vi "lvEtherbone.error_handler.vi"(2 "eb_status":T1, 5 "error in":errorcluster) -> (19 "error out":errorcluster)   [LabVIEW 2009, in "lvEtherbone.lvlib"]
doc: "Builds an error cluster depending on \"eb_status\" and call chain"
uses:
  lvEtherbone.lvlib
  lvEtherbone.lveb_status_t.ctl
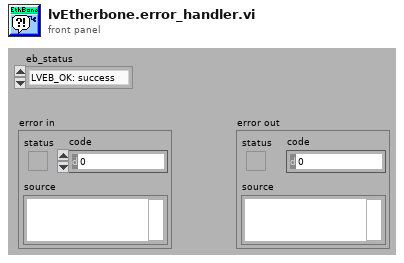
[diagram p1: front panel]
types:
  T1 = typedef "lvEtherbone.lvlib/lvEtherbone.lveb_status_t.ctl" = enum32{"LVEB_OK: success", "LVEB_UNKNOWN: unknown error", "LVEB_OS: operating system forbids access", "LVEB_PORT: port in use or unavailable", "LVEB_ID: ID invalid or out of resources", "LVEB_SOCKET: socket invalid or unavailable", "LVEB_EB: remote address is not Etherbone conformant", "LVEB_IP: bad format or network address", "LVEB_BUSWIDTH: bus width error", "LVEB_DEVICEBUSY: Whishbone device still busy", "LVEB_DEVICEFAIL: operation on Wishbone device failed", "LVEB_DEVICEEXIST: Whishbone device already exists, overlaps, or does not exist", "LVEB_TIMEDOUT: a timeout occurred", "LVEB_OVERFLOW: payload of Etherbone exceeded", "LVEB_ADDRESS: bad address"}
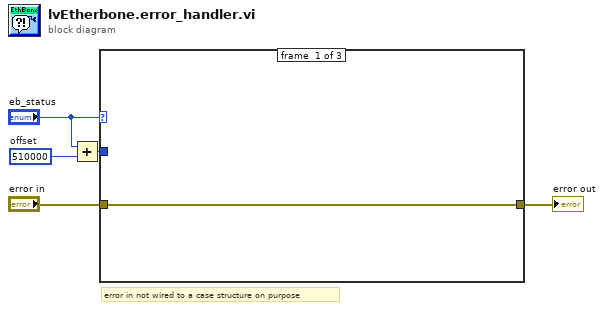
[diagram p0: block diagram]
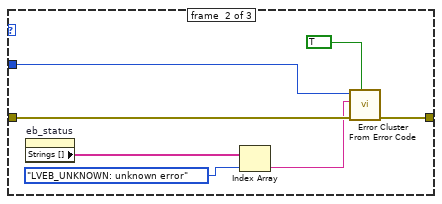
[diagram p2: hidden frame]
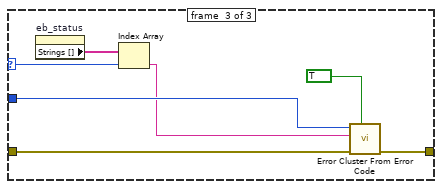
[diagram p3: hidden frame]
diagram:
  w2 = 510000  # offset
  # "error in not wired to a case structure on purpose"
  n1 = Add(x="eb_status", y=w2) -> (x+y=w1:u32)
  n2 = case shown="\"LVEB_UNKNOWN: unknown error\", Default" "eb_status" {
    selector: "eb_status" -> [_ _ w15]
    tunnel: "error in" -> [w6 w10 w18]
    tunnel: [w6 w12 w19] -> w5
    tunnel: w1 -> [_ w11 w17]
    frame #0 {
    }
    frame #1 {
      n3 = property on="eb_status" class="Enum (strict)"() -> ("Strings []"=w9:string[])  [unwired: 2 in, 2 out]
      n4 = Index Array(array=w9, index=lvEtherbone.lveb_status_t."LVEB_UNKNOWN: unknown error" ("eb_status")) -> (element=w7:string)
      n5 = call <vilib>:"Error Cluster From Error Code.vi"("show call chain? (False)"=TRUE, "error in (no error)"=w10, "error message (\"\")"=w7, "error code (0)"=w11) -> ("error out"=w12:errorcluster)  [unwired: 5 in]
    }
    frame #2 {
      n6 = property on="eb_status" class="Enum (strict)"() -> ("Strings []"=w16:string[])  [unwired: 2 in, 2 out]
      n7 = Index Array(array=w16, index=w15) -> (element=w14:string)
      n8 = call <vilib>:"Error Cluster From Error Code.vi"("show call chain? (False)"=TRUE, "error in (no error)"=w18, "error message (\"\")"=w14, "error code (0)"=w17) -> ("error out"=w19:errorcluster)  [unwired: 5 in]
    }
  }
  "error out" <- w5
